vi "Eds Get Image camera1.vi"() -> (2 "Image":T1(plugin-control))   [LabVIEW 2012]
panel:
  in  "ICImagingControl":refnum<k7>(container)
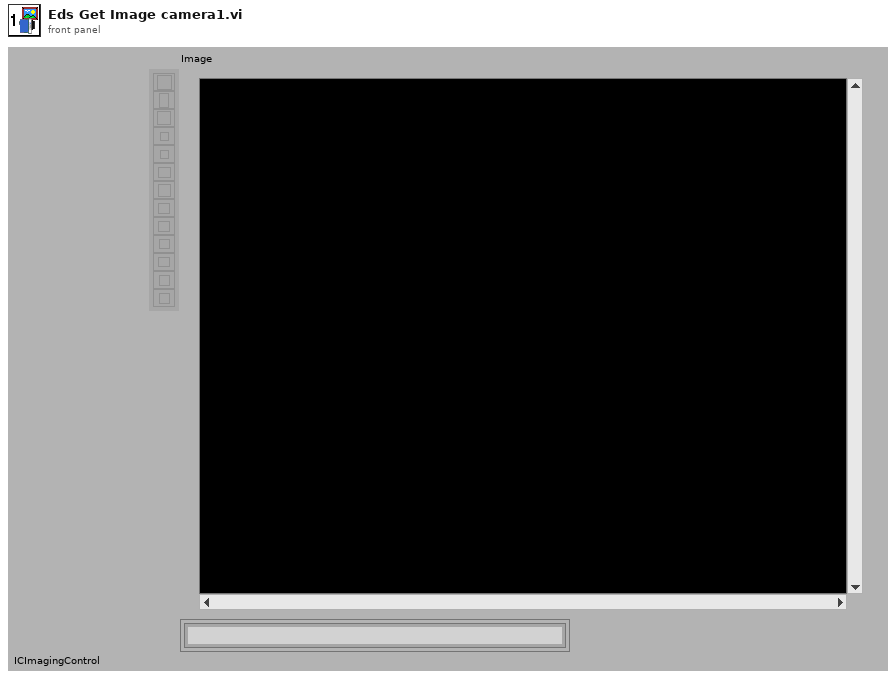
[diagram p1: front panel]
types:
  T1 = typedef "IMAQ Image.ctl" = refnum<image>
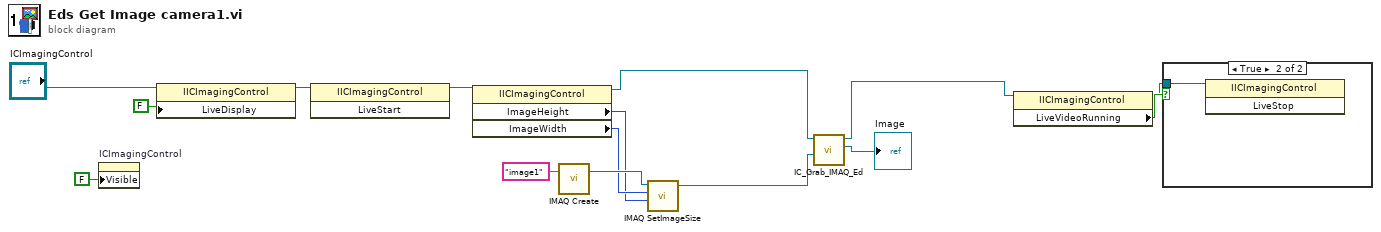
[diagram p0: block diagram]
diagram:
  n1 = property on="ICImagingControl" class="AXCont"("Visible"=FALSE) -> ()  [unwired: 2 in, 2 out]
  n2 = property class="IICImagingControl"(reference="ICImagingControl", "LiveDisplay"=FALSE) -> (reference out=w13:refnum<k7>)  [unwired: 1 in, 1 out]
  n3 = invoke class="IICImagingControl" method="LiveStart"(reference=w13) -> (reference out=w10:refnum<k7>)  [unwired: 2 in, 2 out]
  n4 = property class="IICImagingControl"(reference=w10) -> (reference out=w9:refnum<k7>, "ImageHeight"=w5:i32, "ImageWidth"=w6:i32)  [unwired: 1 in, 1 out]
  n5 = call "IMAQ Create"("Image Name"="image1") -> ("New Image"=w7:T1)  [unwired: 4 in, 1 out]
  n6 = call "IMAQ SetImageSize"("Y Resolution"=w5, "X Resolution"=w6, "Image"=w7) -> ("Image Out"=w4:T1)  [unwired: 2 in, 1 out]
  n7 = call "IC_Grab_IMAQ_Ed.vi"("Image Dest"=w4, "ICImagingControl In"=w9) -> ("Image Out"=→"Image":T1, "ICImagingControl Out"=w12:refnum<k7>)  [unwired: 2 in, 2 out]
  n8 = property class="IICImagingControl"(reference=w12) -> (reference out=w11:refnum<k7>, "LiveVideoRunning"=w15:bool)  [unwired: 1 in, 1 out]
  n9 = case shown="True" w15 {
    tunnel: w11 -> [_ w16]
    frame False {
    }
    frame True {
      n10 = invoke class="IICImagingControl" method="LiveStop"(reference=w16) -> ()  [unwired: 2 in, 3 out]
    }
  }
